vi "Check Folder for AutoMenu Usage.vi"(11 "Target":path) -> (2 "Uses AutoMenu?":bool, 3 "Found AutoMenu Config.ini path":path)   [LabVIEW 2019, in "AutoMenuCreator.lvlib"]
doc: "Check if Target Folder uses AutoMenu."
uses:
  AutoMenuCreator.lvlib
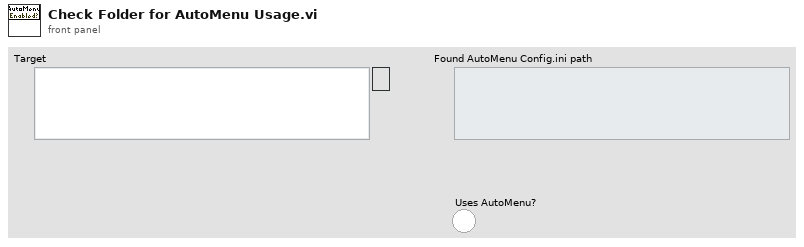
[diagram p1: front panel]
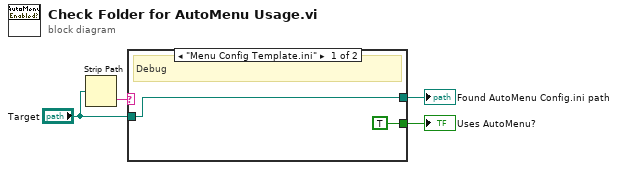
[diagram p0: block diagram]
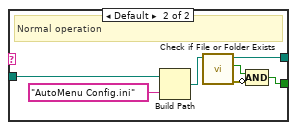
[diagram p2: hidden frame]
diagram:
  n1 = Strip Path(path="Target") -> (name=w1:string)  [unwired: 1 out]
  n2 = case shown="\"Menu Config Template.ini\"" w1 {
    tunnel: [w5 w13] -> w4
    tunnel: [TRUE w10] -> w3
    tunnel: "Target" -> [w5 w8]
    frame "Menu Config Template.ini" {
      # "Debug"
    }
    frame Default {
      # "Normal operation"
      n3 = Build Path(base path=w8, name or relative path="AutoMenu Config.ini") -> (appended path=w11:path)
      n4 = call <vilib>:"Check if File or Folder Exists.vi"("path"=w11) -> ("error out"=w9:errorcluster, "file or folder exists?"=w12:bool, "dup path"=w13:path)  [unwired: 8 in]
      n5 = Compound Arithmetic op=AND(w12, invert w9) -> (w10:bool)
    }
  }
  "Found AutoMenu Config.ini path" <- w4
  "Uses AutoMenu?" <- w3
